vi "Get Instrument Data.vi"(8 "error in (no error)":errorcluster, 9 "Data":dbl[](array[numeric]), 10 "Connection":bool, 11 "Platform in":refnum<class "Platform.lvclass">) -> (0 "error out":errorcluster, 3 "Platform out":refnum<class "Platform.lvclass">)   [LabVIEW 2019, in "Platform.lvlib" / "Platform.lvclass"]
uses:
  Platform.lvclass
  Platform.lvclass/Platform.ctl
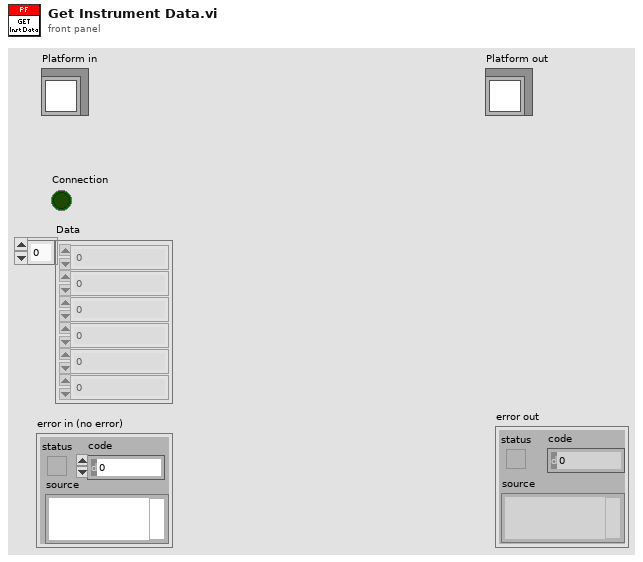
[diagram p1: front panel]
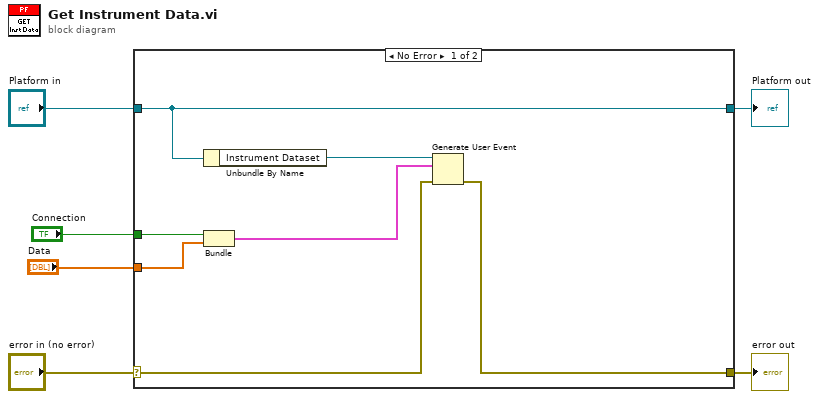
[diagram p0: block diagram]
diagram:
  n1 = case shown="No Error" "error in (no error)" {
    selector: "error in (no error)" -> [w11 w15]
    tunnel: [w10 w15] -> w5
    tunnel: [w13 w14] -> w3
    tunnel: "Platform in" -> [w13 w14]
    tunnel: "Connection" -> [w9 _]
    tunnel: "Data" -> [w8 _]
    frame No Error {
      n2 = Unbundle By Name(w13) -> ("Instrument Dataset"=w12:refnum<user-event>)
      n3 = Bundle("Connection"=w9, "Data"=w8) -> (w7:cluster{"Connection":bool, "Data":dbl[]})  [unwired: 1 in]
      n4 = Generate User Event(user event=w12, event data cluster=w7, error in=w11) -> (error out=w10:errorcluster)  [unwired: 1 in, 1 out]
    }
    frame Error {
    }
  }
  "error out" <- w5
  "Platform out" <- w3
